vi "Longitude dron 1.vi"() -> ()   [LabVIEW 2015, in "Biblioteka moduł map v3.lvlib" / "Zmienne.lvlib" / "Lokalizacja GPS.lvlib"]
uses:
  Lokalizacja GPS.lvlib
panel:
  in  "Longitude dron 1":dbl
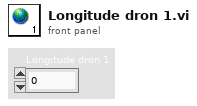
[diagram p1: front panel]
diagram:
